vi "虚拟温度计.vi"() -> ()   [LabVIEW 2018]
panel:
  in  "开关":bool
  out "温度计":dbl(slide) scale=0.0..100.0
  out "电压（mV）":dbl(knob) scale=0.0..1000.0
  # "虚拟温度计"
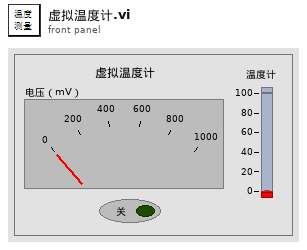
[diagram p1: front panel]
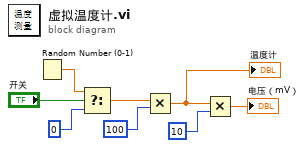
[diagram p0: block diagram]
diagram:
  n1 = Random Number (0-1)() -> (number: 0 to 1=w7:dbl)
  n2 = Select(t=w7, s="开关", f=0) -> (s? t:f=w6:dbl)
  n3 = Multiply(x=w6, y=100) -> (x*y=w2:dbl)
  "温度计" <- w2
  n4 = Multiply(x=w2, y=10) -> (x*y=→"电压（mV）":dbl)
